vi "SetDataString.vi"(8 "error in (no error)":errorcluster, 10 "DataString":string, 11 "FolloWin in":refnum<class "FolloWin.lvclass">) -> (0 "error out":errorcluster, 3 "FolloWin out":refnum<class "FolloWin.lvclass">)   [LabVIEW 2023, in "FolloWin.lvclass"]
doc: "Updates the DataString in FolloWin"
uses:
  FolloWin.lvclass
  FolloWin.lvclass/FolloWin.ctl
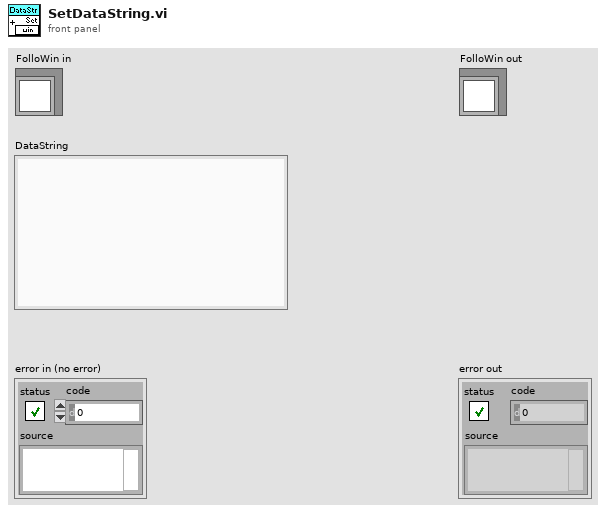
[diagram p1: front panel]
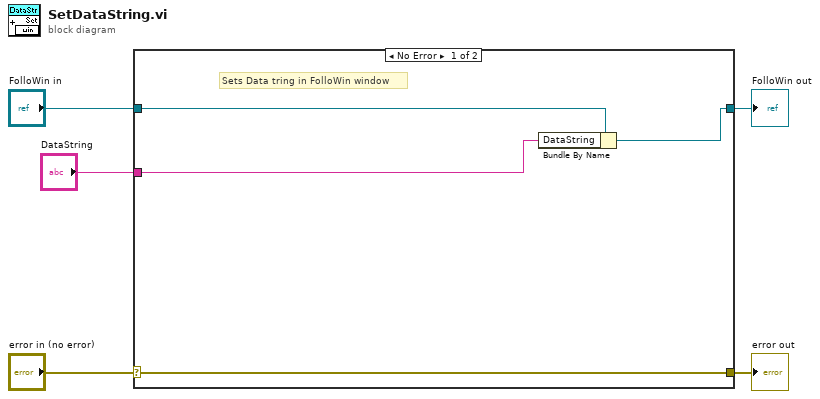
[diagram p0: block diagram]
diagram:
  n1 = case shown="No Error" "error in (no error)" {
    selector: "error in (no error)" -> [w6 w11]
    tunnel: [w6 w11] -> w4
    tunnel: [w8 w10] -> w2
    tunnel: "FolloWin in" -> [w9 w10]
    tunnel: "DataString" -> [w7 _]
    frame No Error {
      # "Sets Data tring in FolloWin window"
      n2 = Bundle By Name(cluster=w9, "DataString"=w7) -> (w8:refnum<class "FolloWin.lvclass">)
    }
    frame Error {
    }
  }
  "error out" <- w4
  "FolloWin out" <- w2
